vi "PID Table (IMC - First Order).vi"(5 "Integrator ?":bool, 6 "Desired Time Constant (tau_c)":dbl, 7 "Type of Controller":u16(ring) items=["P", "PI", "PID"], 9 "Plant delay (theta)":dbl, 10 "Plant time constant (tau)":dbl, 11 "Plant gain (K)":dbl) -> (1 "TD":dbl, 2 "Ti":dbl, 3 "Kc":dbl)   [LabVIEW 2020, in "NI_PID_autopid.lvlib"]
uses:
  <vilib>/addons/control/pid/NI_PID_autopid.lvlib
panel:
  # "Plant Parameters"
  # "Specs"
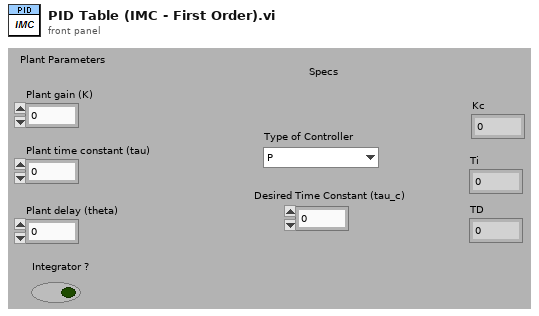
[diagram p1: front panel]
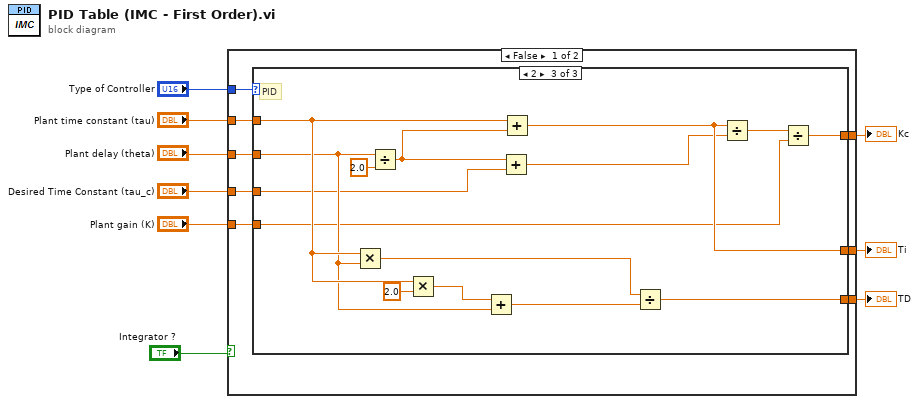
[diagram p0: block diagram]
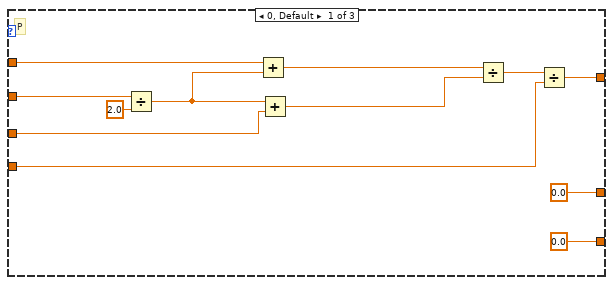
[diagram p2: hidden frame]
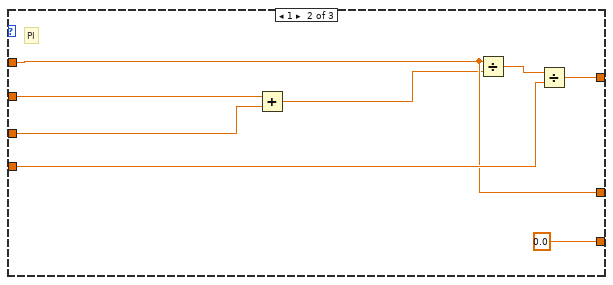
[diagram p3: hidden frame]
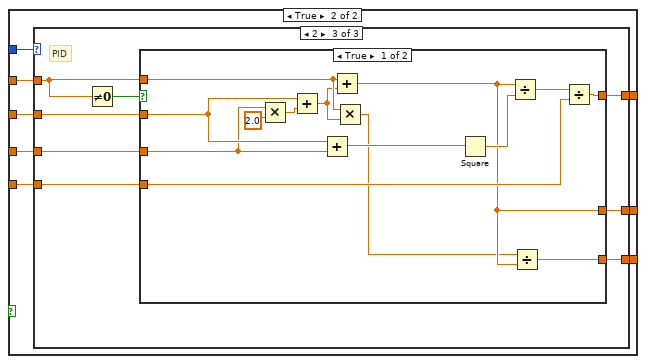
[diagram p4: hidden frame]
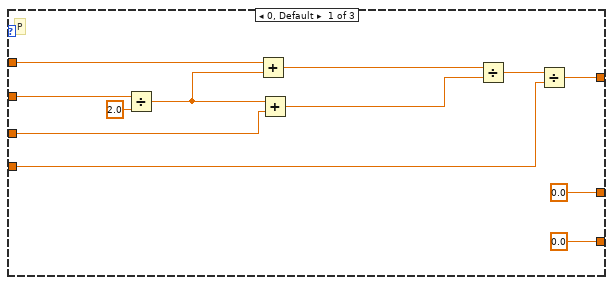
[diagram p5: hidden frame]
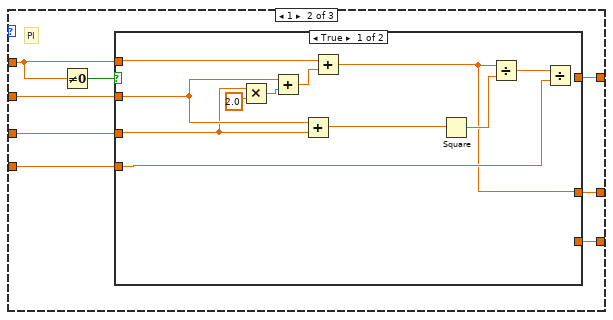
[diagram p6: hidden frame]
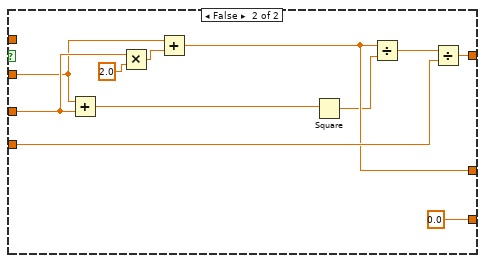
[diagram p7: hidden frame]
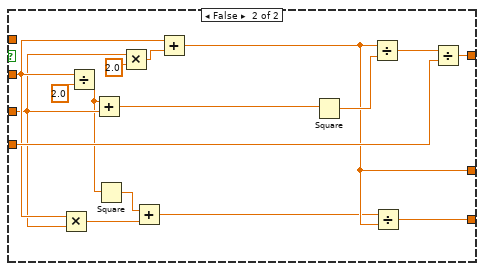
[diagram p8: hidden frame]
diagram:
  n1 = case shown="False" "Integrator ?" {
    tunnel: "Plant time constant (tau)" -> [w17 w60]
    tunnel: "Plant delay (theta)" -> [w16 w59]
    tunnel: [w15 w58] -> w7
    tunnel: [w14 w57] -> w6
    tunnel: "Desired Time Constant (tau_c)" -> [w13 w56]
    tunnel: [w12 w55] -> w4
    tunnel: "Type of Controller" -> [w11 w54]
    tunnel: "Plant gain (K)" -> [w10 w53]
    frame False {
      n2 = case shown="2" w11 {
        tunnel: w17 -> [w28 w32 w51]
        tunnel: w16 -> [w25 w34 w48]
        tunnel: [0.0 0.0 w47] -> w15
        tunnel: [0.0 w32 w46] -> w14
        tunnel: w13 -> [w21 w33 w45]
        tunnel: [w19 w36 w43] -> w12
        tunnel: w10 -> [w18 w35 w38]
        frame 0, Default {
          # "P"
          n3 = Divide(x=w25, y=2.0) -> (x/y=w27:dbl)
          n4 = Add(x=w28, y=w27) -> (x+y=w23:dbl)
          n5 = Add(x=w27, y=w21) -> (x+y=w20:dbl)
          n6 = Divide(x=w23, y=w20) -> (x/y=w26:dbl)
          n7 = Divide(x=w26, y=w18) -> (x/y=w19:dbl)
        }
        frame 1 {
          # "PI"
          n8 = Add(x=w34, y=w33) -> (x+y=w30:dbl)
          n9 = Divide(x=w32, y=w30) -> (x/y=w31:dbl)
          n10 = Divide(x=w31, y=w35) -> (x/y=w36:dbl)
        }
        frame 2 {
          # "PID"
          n11 = Multiply(x=w51, y=w48) -> (x*y=w40:dbl)
          n12 = Divide(x=w48, y=2.0) -> (x/y=w50:dbl)
          n13 = Multiply(x=w51, y=2.0) -> (x*y=w41:dbl)
          n14 = Add(x=w41, y=w48) -> (x+y=w39:dbl)
          n15 = Add(x=w50, y=w45) -> (x+y=w44:dbl)
          n16 = Add(x=w51, y=w50) -> (x+y=w46:dbl)
          n17 = Divide(x=w40, y=w39) -> (x/y=w47:dbl)
          n18 = Divide(x=w46, y=w44) -> (x/y=w49:dbl)
          n19 = Divide(x=w49, y=w38) -> (x/y=w43:dbl)
        }
      }
    }
    frame True {
      n20 = case shown="2" w54 {
        tunnel: w60 -> [w71 w73 w103]
        tunnel: w59 -> [w68 w77 w107]
        tunnel: [0.0 w80 w110] -> w58
        tunnel: [0.0 w76 w106] -> w57
        tunnel: w56 -> [w64 w75 w105]
        tunnel: [w62 w79 w109] -> w55
        tunnel: w53 -> [w61 w78 w108]
        frame 0, Default {
          # "P"
          n21 = Divide(x=w68, y=2.0) -> (x/y=w70:dbl)
          n22 = Add(x=w71, y=w70) -> (x+y=w66:dbl)
          n23 = Add(x=w70, y=w64) -> (x+y=w63:dbl)
          n24 = Divide(x=w66, y=w63) -> (x/y=w69:dbl)
          n25 = Divide(x=w69, y=w61) -> (x/y=w62:dbl)
        }
        frame 1 {
          # "PI"
          n26 = Not Equal To 0?(x=w73) -> (x != 0?=w74:bool)
          n27 = case shown="True" w74 {
            tunnel: [_ 0.0] -> w80
            tunnel: [_ w100] -> w79
            tunnel: w78 -> [w82 w99]
            tunnel: w77 -> [w84 w94]
            tunnel: [w81 w97] -> w76
            tunnel: w75 -> [w83 w95]
            tunnel: w73 -> [w85 _]
            frame True {
              n28 = Multiply(x=w83, y=2.0) -> (x*y=w90:dbl)
              n29 = Add(x=w84, y=w90) -> (x+y=w86:dbl)
              n30 = Add(x=w84, y=w83) -> (x+y=w88:dbl)
              n31 = Add(x=w85, y=w86) -> (x+y=w81:dbl)
              n32 = Square(x=w88) -> (x^2=w87:dbl)
              n33 = Divide(x=w81, y=w87) -> (x/y=w91:dbl)
              n34 = Divide(x=w91, y=w82) -> ()  [unwired: 1 out]
            }
            frame False {
              n35 = Add(x=w94, y=w95) -> (x+y=w93:dbl)
              n36 = Multiply(x=w95, y=2.0) -> (x*y=w96:dbl)
              n37 = Add(x=w94, y=w96) -> (x+y=w97:dbl)
              n38 = Square(x=w93) -> (x^2=w92:dbl)
              n39 = Divide(x=w97, y=w92) -> (x/y=w102:dbl)
              n40 = Divide(x=w102, y=w99) -> (x/y=w100:dbl)
            }
          }
        }
        frame 2 {
          # "PID"
          n41 = Not Equal To 0?(x=w103) -> (x != 0?=w104:bool)
          n42 = case shown="True" w104 {
            tunnel: [w113 w125] -> w110
            tunnel: [w123 w139] -> w109
            tunnel: w108 -> [w122 w138]
            tunnel: w107 -> [w118 w132]
            tunnel: [w112 w127] -> w106
            tunnel: w105 -> [w117 w131]
            tunnel: w103 -> [w115 _]
            frame True {
              n43 = Multiply(x=w117, y=2.0) -> (x*y=w121:dbl)
              n44 = Add(x=w118, y=w121) -> (x+y=w114:dbl)
              n45 = Add(x=w118, y=w117) -> (x+y=w119:dbl)
              n46 = Add(x=w115, y=w114) -> (x+y=w112:dbl)
              n47 = Multiply(x=w115, y=w114) -> (x*y=w111:dbl)
              n48 = Square(x=w119) -> (x^2=w116:dbl)
              n49 = Divide(x=w112, y=w116) -> (x/y=w124:dbl)
              n50 = Divide(x=w111, y=w112) -> (x/y=w113:dbl)
              n51 = Divide(x=w124, y=w122) -> (x/y=w123:dbl)
            }
            frame False {
              n52 = Multiply(x=w132, y=w131) -> (x*y=w130:dbl)
              n53 = Divide(x=w132, y=2.0) -> (x/y=w129:dbl)
              n54 = Add(x=w129, y=w131) -> (x+y=w135:dbl)
              n55 = Square(x=w129) -> (x^2=w128:dbl)
              n56 = Multiply(x=w131, y=2.0) -> (x*y=w136:dbl)
              n57 = Add(x=w128, y=w130) -> (x+y=w126:dbl)
              n58 = Add(x=w132, y=w136) -> (x+y=w127:dbl)
              n59 = Square(x=w135) -> (x^2=w134:dbl)
              n60 = Divide(x=w127, y=w134) -> (x/y=w140:dbl)
              n61 = Divide(x=w126, y=w127) -> (x/y=w125:dbl)
              n62 = Divide(x=w140, y=w138) -> (x/y=w139:dbl)
            }
          }
        }
      }
    }
  }
  "Kc" <- w4
  "Ti" <- w6
  "TD" <- w7
